vi "create data log.vi"(0 "Header String":string="This is a log file of a temperture control run being done in Physics 350. It records the temperature, power, the control bandwidth, and settle bandwidth parameters versus time.", 11 "error in":errorcluster) -> (4 "cancelled":bool=TRUE, 8 "file refnum out":refnum<file>, 15 "error out":errorcluster)   [LabVIEW 2016]
doc: "This vi prompts the user to choose whether to create a data log. If the user indicates to the affirmative, a log file is created with a given header.\n\nPaul K Dixon\nPhysics 350\nCSUSB Physics"
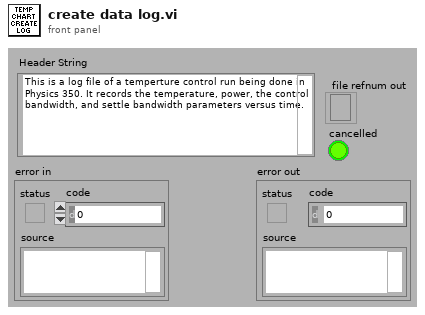
[diagram p1: front panel]
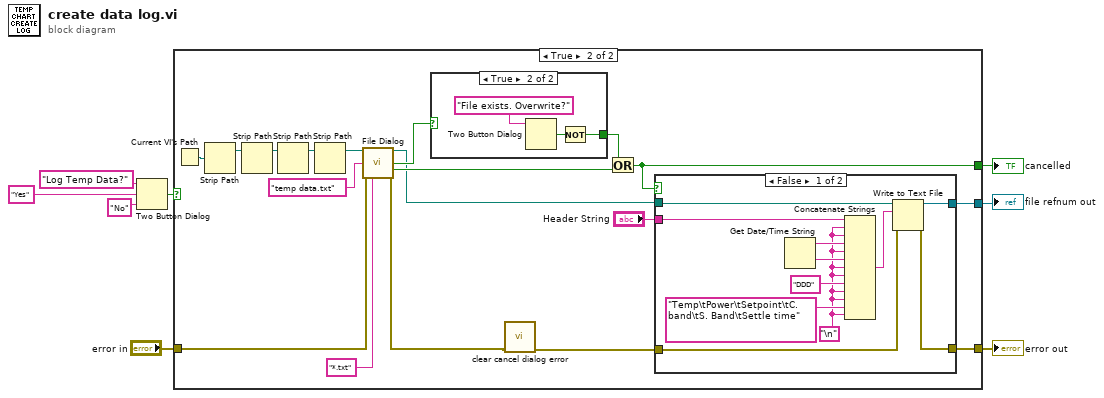
[diagram p0: block diagram]
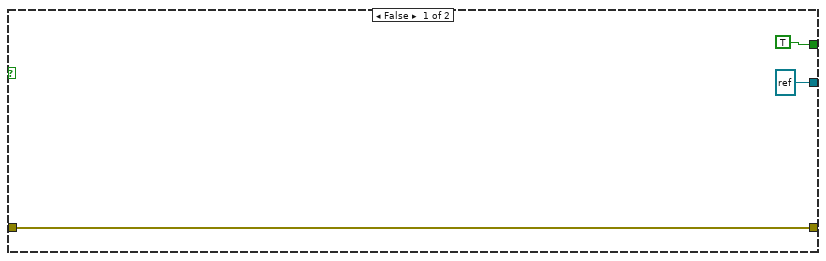
[diagram p2: hidden frame]
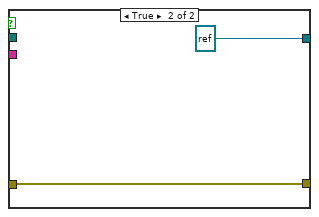
[diagram p3: hidden frame]
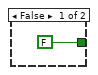
[diagram p4: hidden frame]
diagram:
  n1 = Two Button Dialog(message="Log Temp Data?", 1:"No" ("F button name (\"Cancel\")"), 2:"Yes" ("T button name (\"OK\")")) -> (T button?=w2:bool)
  n2 = case shown="True" w2 {
    tunnel: [TRUE w25] -> w8
    tunnel: [w11 w23] -> w7
    tunnel: [refnum<file> refnum ("refnum out") w22] -> w6
    tunnel: "error in" -> [w11 w17]
    frame False {
    }
    frame True {
      n3 = Current VI's Path() -> (path=w28:path)
      n4 = Strip Path(path=w28) -> (stripped path=w29:path)  [unwired: 1 out]
      n5 = Strip Path(path=w29) -> (stripped path=w21:path)  [unwired: 1 out]
      n6 = Strip Path(path=w21) -> (stripped path=w20:path)  [unwired: 1 out]
      n7 = Strip Path(path=w20) -> (stripped path=w16:path)  [unwired: 1 out]
      n8 = call "File Dialog"("start path"=w16, "default name"="temp data.txt" ("name or relative path"), "error in"=w17, "pattern (all files)"="*.txt") -> ("selected path"=w13:path, "exists"=w15:bool, "cancelled"=w14:bool, "error out"=w12:errorcluster)  [unwired: 8 in]
      n9 = case shown="True" w15 {
        tunnel: [FALSE ("T button?") w44] -> w27
        frame False {
        }
        frame True {
          n10 = Two Button Dialog(message="File exists. Overwrite?") -> (T button?=w45:bool)  [unwired: 2 out]
          n11 = Not(x=w45) -> (.not. x?=w44:bool)
        }
      }
      n12 = call "clear cancel dialog error.vi"("error in"=w12) -> ("error out"=w24:errorcluster)  [unwired: 14 out]
      n13 = Or(x=w27, y=w14) -> (x .or. y?=w25:bool)
      n14 = case shown="False" w25 {
        tunnel: "Header String" -> [w31 _]
        tunnel: w13 -> [w39 _]
        tunnel: w24 -> [w38 w41]
        tunnel: [w37 w41] -> w23
        tunnel: [w36 refnum<file> refnum ("refnum out")] -> w22
        frame False {
          w30 = "\n"
          n15 = Get Date/Time String() -> (date string=w33:string, time string=w32:string)  [unwired: 3 in]
          n16 = Concatenate Strings(w31, w30, w30, w33, w30, w32, w30, w30, "DDD", w30, w30, "Temp\tPower\tSetpoint\tC. band\tS. Band\tSettle time", w30) -> (w40:string)
          n17 = Write to Text File(file (use dialog)=w39, text=w40, error in=w38) -> (refnum out=w36:refnum<file>, error out=w37:errorcluster)  [unwired: 2 out]
        }
        frame True {
        }
      }
    }
  }
  "cancelled" <- w8
  "error out" <- w7
  "file refnum out" <- w6
